vi "Main FPGA.vi"() -> ()   [LabVIEW 2020]
uses:
  <vilib>/Platform/TimedLoop/XDataNode/timing_clust.ctl
  <vilib>/Platform/TimedLoop/XDataNode/nitl_modes.ctl
  <vilib>/Platform/TimedLoop/XDataNode/wakeup.ctl
  <vilib>/rvi/eio/common/nirviEmuTemplateMethod_errors.vi
  <vilib>/rvi/Emulation/niFpgaGetClockAttributes.vi
  <vilib>/rvi/Emulation/niFpgaSctlEmulationGetInTimedLoop.vi
  <vilib>/rvi/Emulation/niFpgaEmulationReportErrorSimple.vi
  <vilib>/rvi/Emulation/niFpgaCriticalErrorInLSC.vi
  <vilib>/rvi/Emulation/niFpgaProcessEmulError.vi
  <vilib>/rvi/interface/RandomDataEmulation/nirviRandomDataMultiElementFPGAFIFO.vi
  <instcachedir>/0/nirviRandomDataMultiElementFPGAFIFO_3E9965BA1FAD4E7B8DABA31768A09B1F.lvgen/nirviRandomDataMultiElementFPGAFIFO_3E9965BA1FAD4E7B8DABA31768A09B1F_001.vi
  <vilib>/rvi/interface/RandomDataEmulation/niFpgaRandomDataHandleErrors.vi
  <vilib>/eio/EIOMethodNode/EIOMethodNode.xnode
  <vilib>/eio/EIONode/EIONode.xnode
  <vilib>/rvi/DataTransferAndStorage/Container/XNode/niFpgaContainer.xnode
  <vilib>/rvi/interface/RandomDataEmulation/nirviRandomDataFpgaMultiElementTemplate.vi
  <vilib>/Platform/TimedLoop/XDataNode/XDataNode.xnode
  <vilib>/Platform/TimedLoop/XDataNode/XDNodeRunTimeDep.lvlib
panel:
  out "Vgen":fxp<+/-,20,5>
  out "Numeric":i32
  out "Timed Out?":bool
  in  "STOP SCTL":bool
  in  "Fase PWM Corrientes":fxp<+,32,0>
  out "Relé encendido":bool
  in  "Fase PWM voltajes":fxp<+,32,0>
  in  "Inc. Fase Volt.":fxp<+,27,0>=0.00020000338554382324
  in  "Freq PWM Corr.":fxp<+,32,0>=0.0005000000819563866
  in  "Freq. PWM Volt.":fxp<+,32,0>=0.0005000000819563866
  in  "Modulacion T002":fxp<+/-,16,1>
  in  "Modulacion T001":fxp<+/-,16,1>
  in  "Factor de Ajuste U1":fxp<+/-,32,2>=1.0
  in  "Factor de Ajuste V1":fxp<+/-,32,2>=0.9900000002235174
  in  "Factor de Ajuste W1":fxp<+/-,32,2>=0.9720000000670552
  in  "Factor de Ajuste U3":fxp<+/-,32,2>=0.9840000001713634
  in  "Factor de Ajuste V3":fxp<+/-,32,2>=0.9840000001713634
  in  "Factor de Ajuste W3":fxp<+/-,32,2>=0.9840000001713634
  out "W4 - U4":fxp<+/-,17,3>
  out "V4 - W4":fxp<+/-,17,3>
  out "U4 - V4":fxp<+/-,17,3>
  out "W3 - U3":fxp<+/-,17,3>
  out "V3 - W3":fxp<+/-,17,3>
  out "U3 - V3":fxp<+/-,17,3>
  out "W2 - U2":fxp<+/-,17,3>
  out "V2 - W2":fxp<+/-,17,3>
  out "U2 - V2":fxp<+/-,17,3>
  out "W1 - U1":fxp<+/-,17,3>
  out "V1 - W1":fxp<+/-,17,3>
  out "U1 - V1":fxp<+/-,17,3>
  in  "Falla U4":bool
  in  "Falla W4":bool
  in  "Falla U3":bool
  in  "Falla W3":bool
  in  "Falla W2":bool
  in  "Falla U2":bool
  in  "Falla W1":bool
  in  "Amplitud Corrientes":fxp<+,32,0>
  in  "Falla U1":bool
  out "sin x + 270":fxp<+/-,16,2>
  out "sin x + 285":fxp<+/-,16,2>
  out "sin x + 165":fxp<+/-,16,2>
  out "sin x + 45":fxp<+/-,16,2>
  out "sin x + 135":fxp<+/-,16,2>
  out "sin x + 150":fxp<+/-,16,2>
  out "sin x + 30":fxp<+/-,16,2>
  out "sin x + 255":fxp<+/-,16,2>
  out "sin x + 15":fxp<+/-,16,2>
  out "sin x + 240":fxp<+/-,16,2>
  out "sin x + 120":fxp<+/-,16,2>
  in  "Phase Inc Corriente":fxp<+,27,0>=0.00010000169277191162
  out "sin(x)":fxp<+/-,16,2>
  in  "Stop While":bool
  out "IExc":fxp<+/-,20,5>
  # "Control PWM de Voltajes"
  # "Importante, para detener la ejecución presionar estos dos botones de STOP"
  # "frecuencia PWM corrientes"
  # "20 kHz / 40 MHz = 0,0005 periods/tick"
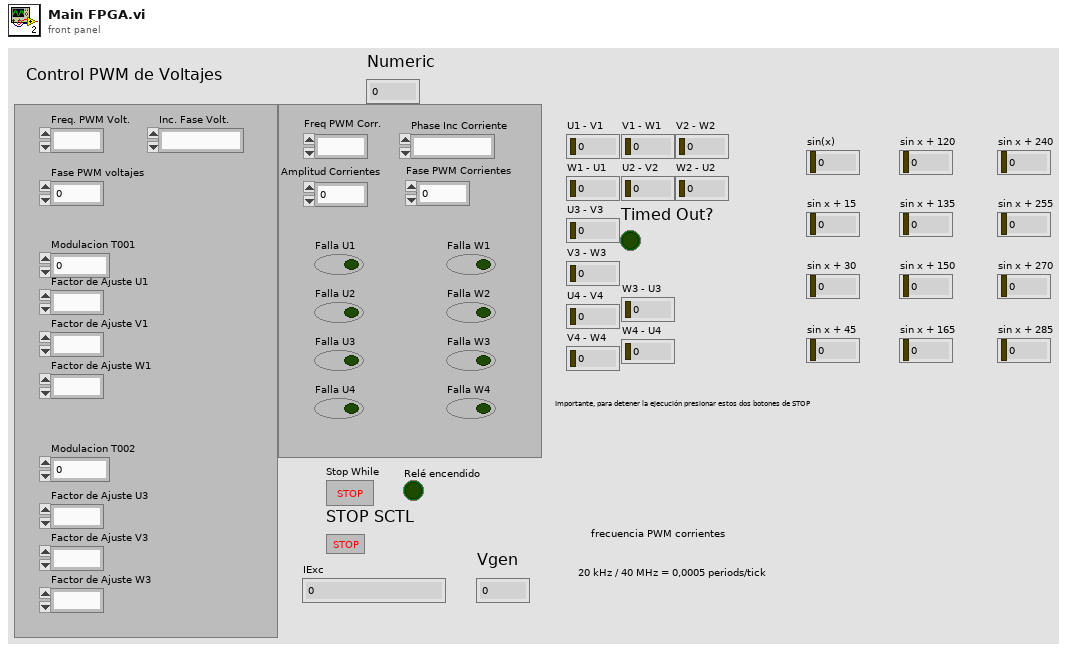
[diagram p1: front panel]
types:
  T1 = typedef "XDNodeRunTimeDep.lvlib/timing_clust.ctl" = cluster{"Expected End [f-1]":u64, "Actual End [f-1]":u64, "Finished Late? [f-1]":bool, "Expected End [i-1]":u64, "Actual End [i-1]":u64, "Finished Late? [i-1]":bool, "Expected Start [i]":u64, "Actual Start [i]":u64, "Expected Start [f]":u64, "Actual Start [f]":u64, "Source Name":string, "Structure Name":string, "Period":i64, "Deadline":i64, "Offset":i64, "Start":i64, "Priority":i32, "Timeout":i32, "Mode":T2, "Wakeup Reason":T3, "Error":errorcluster, "Source Type":string, "Secondary Source Type":string, "Global End Time":u64, "Global Start Time":u64, "Frame Duration":u64, "Iteration Duration":u64, "Assigned CPU":i32, "I/O Scan Engine Mode":u32}
  T2 = typedef "XDNodeRunTimeDep.lvlib/nitl_modes.ctl" = enum32{"No Change", "Process missed periods, maintain original phase", "Discard missed periods, maintain original phase", "Process missed periods, ignore original phase", "Discard missed periods, ignore original phase"}
  T3 = typedef "XDNodeRunTimeDep.lvlib/wakeup.ctl" = enum32{"Normal", "Aborted", "Asynchronous wakeup", "Timing source error", "Timed loop error", "Timeout"}
  T4 = cluster{"U1 - V1":fxp<+/-,17,3>, "V1 - W1":fxp<+/-,17,3>, "W1 - U1":fxp<+/-,17,3>, "U2 - V2":fxp<+/-,17,3>, "V2 - W2":fxp<+/-,17,3>, "W2 - U2":fxp<+/-,17,3>, "U3 - V3":fxp<+/-,17,3>, "V3 - W3":fxp<+/-,17,3>, "W3 - U3":fxp<+/-,17,3>, "U4 - V4":fxp<+/-,17,3>, "V4 - W4":fxp<+/-,17,3>, "W4 - U4":fxp<+/-,17,3>}
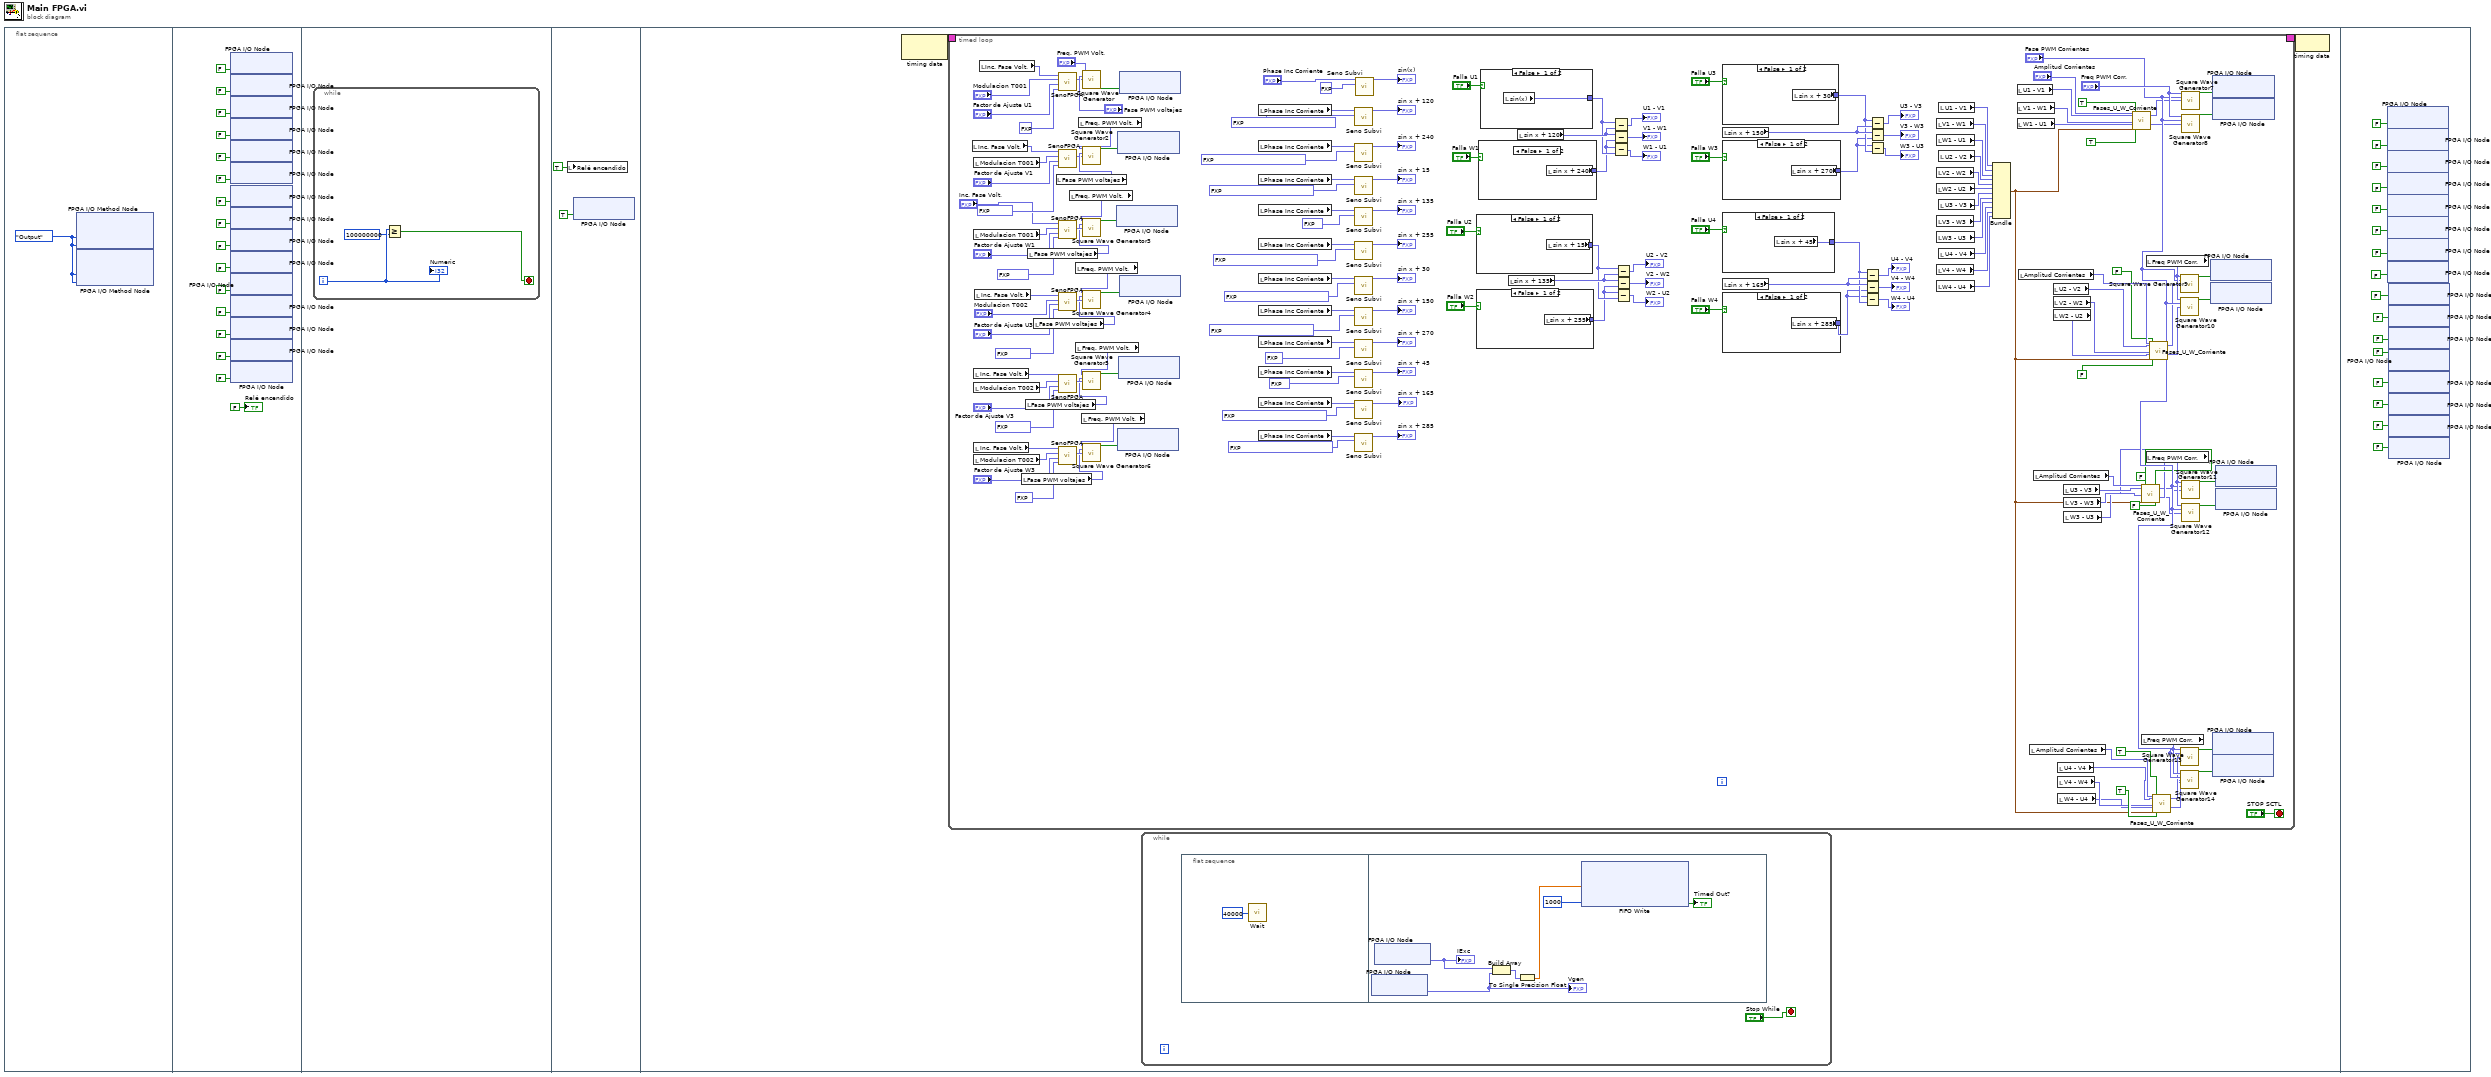
[diagram p0: block diagram]
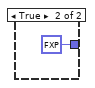
[diagram p2: hidden frame]
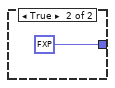
[diagram p3: hidden frame]
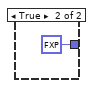
[diagram p4: hidden frame]
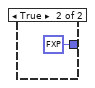
[diagram p5: hidden frame]
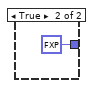
[diagram p6: hidden frame]
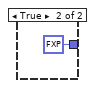
[diagram p7: hidden frame]
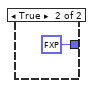
[diagram p8: hidden frame]
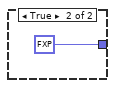
[diagram p9: hidden frame]
diagram:
  n1 = flat-sequence {
    frame #0 {
      w1 = enum8{"No Change", "Input", "Output"}."Output" ("DIO 7:4")
      n2 = xnode "FPGA I/O Method Node"("DIO 7:4"=w1, "DIO 3:0"=w1) -> ()  [unwired: 1 in, 1 out]
      n3 = xnode "FPGA I/O Method Node"("DIO 7:4"=w1, "DIO 3:0"=w1) -> ()  [unwired: 1 in, 1 out]
    }
    frame #1 {
      n4 = xnode "FPGA I/O Node"("Mod1/DIO0"=FALSE) -> ()  [unwired: 1 in, 1 out]
      n5 = xnode "FPGA I/O Node"("Mod1/DIO1"=FALSE) -> ()  [unwired: 1 in, 1 out]
      n6 = xnode "FPGA I/O Node"("Mod1/DIO2"=FALSE) -> ()  [unwired: 1 in, 1 out]
      n7 = xnode "FPGA I/O Node"("Mod1/DIO4"=FALSE ("Mod1/DIO3")) -> ()  [unwired: 1 in, 1 out]
      n8 = xnode "FPGA I/O Node"("Mod1/DIO5"=FALSE ("Mod1/DIO4")) -> ()  [unwired: 1 in, 1 out]
      n9 = xnode "FPGA I/O Node"("Mod1/DIO6"=FALSE ("Mod1/DIO0")) -> ()  [unwired: 1 in, 1 out]
      n10 = xnode "FPGA I/O Node"("Mod1/DIO7"=FALSE ("Mod1/DIO3")) -> ()  [unwired: 1 in, 1 out]
      n11 = xnode "FPGA I/O Node"("Mod2/DIO0"=FALSE ("Mod1/DIO3")) -> ()  [unwired: 1 in, 1 out]
      n12 = xnode "FPGA I/O Node"("Mod2/DIO1"=FALSE ("Mod1/DIO4")) -> ()  [unwired: 1 in, 1 out]
      n13 = xnode "FPGA I/O Node"("Mod2/DIO2"=FALSE ("Mod1/DIO3")) -> ()  [unwired: 1 in, 1 out]
      n14 = xnode "FPGA I/O Node"("Mod2/DIO3"=FALSE ("Mod1/DIO4")) -> ()  [unwired: 1 in, 1 out]
      n15 = xnode "FPGA I/O Node"("Mod2/DIO4"=FALSE ("Mod1/DIO3")) -> ()  [unwired: 1 in, 1 out]
      n16 = xnode "FPGA I/O Node"("Mod2/DIO5"=FALSE ("Mod1/DIO4")) -> ()  [unwired: 1 in, 1 out]
      n17 = xnode "FPGA I/O Node"("Mod2/DIO6"=FALSE ("Mod1/DIO4")) -> ()  [unwired: 1 in, 1 out]
      n18 = xnode "FPGA I/O Node"("Mod2/DIO7"=FALSE ("Mod1/DIO3")) -> ()  [unwired: 1 in, 1 out]
      "Relé encendido" <- FALSE ("Relé encendido")
    }
    frame #2 {
      n19 = while {
        i -> [w20]
        stop <- w18 stop-if-true
        n20 = Greater Or Equal?(x=w20, y=100000000) -> (x >= y?=w18:bool)
        "Numeric" <- w20
      }
    }
    frame #3 {
      n21 = local write "Relé encendido"(TRUE ("Relé encendido")) -> ()
      n22 = xnode "FPGA I/O Node"("Mod1/DIO7"=TRUE ("Mod1/DIO0")) -> ()  [unwired: 1 in, 1 out]
    }
    frame #4 {
      n23 = node-c288() -> (w24:T1)  [unwired: 1 in]
      n24 = timed-loop {
        timing: w24 -> [_]
        timing-out: [_] -> w23
        stop <- "STOP SCTL" stop-if-true
        n25 = local read "Inc. Fase Volt."() -> (w34:fxp<+,27,0>)
        n26 = local read "Modulacion T001"() -> (w110:fxp<+/-,16,1>)
        n27 = local read "Modulacion T001"() -> (w113:fxp<+/-,16,1>)
        n28 = local read "Inc. Fase Volt."() -> (w89:fxp<+,27,0>)
        n29 = local read "Modulacion T002"() -> (w120:fxp<+/-,16,1>)
        n30 = local read "Inc. Fase Volt."() -> (w88:fxp<+,27,0>)
        n31 = local read "Modulacion T002"() -> (w124:fxp<+/-,16,1>)
        n32 = local read "Inc. Fase Volt."() -> (w90:fxp<+,27,0>)
        n33 = local read "Inc. Fase Volt."() -> (w35:fxp<+,27,0>)
        n34 = local read "Fase PWM voltajes"() -> (w74:fxp<+,32,0>)
        n35 = local read "Fase PWM voltajes"() -> (w75:fxp<+,32,0>)
        n36 = local read "Fase PWM voltajes"() -> (w77:fxp<+,32,0>)
        n37 = local read "Fase PWM voltajes"() -> (w76:fxp<+,32,0>)
        n38 = local read "Fase PWM voltajes"() -> (w78:fxp<+,32,0>)
        n39 = call "SenoFPGA.vi"("Fase Inicial"=fxp<+,27,1> 0.0 ("Fase Inicial U1"), "Factor de Ajuste"="Factor de Ajuste U1", "Modulacion T001"="Modulacion T001", "Tasa de Incremento de Fase"=w35) -> ("Sine Wave"=w38:fxp<+/-,32,2>)  [unwired: 7 in]
        n40 = call "SenoFPGA.vi"("Fase Inicial"=fxp<+,27,1> 0.6666666567325592 ("Fase Inicial V1"), "Factor de Ajuste"="Factor de Ajuste V1", "Modulacion T001"=w110, "Tasa de Incremento de Fase"=w34) -> ("Sine Wave"=w37:fxp<+/-,32,2>)  [unwired: 7 in]
        n41 = call "SenoFPGA.vi"("Fase Inicial"=fxp<+,27,1> 1.3333333283662796 ("Fase Inicial W1"), "Factor de Ajuste"="Factor de Ajuste W1", "Modulacion T001"=w113, "Tasa de Incremento de Fase"="Inc. Fase Volt.") -> ("Sine Wave"=w114:fxp<+/-,32,2>)  [unwired: 7 in]
        n42 = call "SenoFPGA.vi"("Fase Inicial"=fxp<+,27,1> 0.16666659712791443 ("Fase Inicial U3"), "Factor de Ajuste"="Factor de Ajuste U3", "Modulacion T001"="Modulacion T002", "Tasa de Incremento de Fase"=w90) -> ("Sine Wave"=w117:fxp<+/-,32,2>)  [unwired: 7 in]
        n43 = call "SenoFPGA.vi"("Fase Inicial"=fxp<+,27,1> 0.8333333283662796 ("Fase Inicial V3"), "Factor de Ajuste"="Factor de Ajuste V3", "Modulacion T001"=w120, "Tasa de Incremento de Fase"=w89) -> ("Sine Wave"=w121:fxp<+/-,32,2>)  [unwired: 7 in]
        n44 = call "SenoFPGA.vi"("Fase Inicial"=fxp<+,27,1> 1.5 ("Fase Inicial W3"), "Factor de Ajuste"="Factor de Ajuste W3", "Modulacion T001"=w124, "Tasa de Incremento de Fase"=w88) -> ("Sine Wave"=w125:fxp<+/-,32,2>)  [unwired: 7 in]
        n45 = local read "Freq. PWM Volt."() -> (w99:fxp<+,32,0>)
        n46 = local read "Freq. PWM Volt."() -> (w98:fxp<+,32,0>)
        n47 = local read "Freq. PWM Volt."() -> (w97:fxp<+,32,0>)
        n48 = local read "Freq. PWM Volt."() -> (w100:fxp<+,32,0>)
        n49 = local read "Freq. PWM Volt."() -> (w96:fxp<+,32,0>)
        n50 = call "Square Wave Generator"("frequency (periods/tick)"="Freq. PWM Volt.", "phase offset (periods)"="Fase PWM voltajes", "duty cycle (periods)"=w38) -> ("square wave out"=w107:bool)  [unwired: 12 in]
        n51 = call "Square Wave Generator2"("frequency (periods/tick)"=w100, "phase offset (periods)"=w78, "duty cycle (periods)"=w37) -> ("square wave out"=w106:bool)  [unwired: 12 in]
        n52 = call "Square Wave Generator3"("frequency (periods/tick)"=w99, "phase offset (periods)"=w77, "duty cycle (periods)"=w114) -> ("square wave out"=w105:bool)  [unwired: 12 in]
        n53 = call "Square Wave Generator4"("frequency (periods/tick)"=w98, "phase offset (periods)"=w76, "duty cycle (periods)"=w117) -> ("square wave out"=w104:bool)  [unwired: 12 in]
        n54 = call "Square Wave Generator5"("frequency (periods/tick)"=w97, "phase offset (periods)"=w75, "duty cycle (periods)"=w121) -> ("square wave out"=w103:bool)  [unwired: 12 in]
        n55 = call "Square Wave Generator6"("frequency (periods/tick)"=w96, "phase offset (periods)"=w74, "duty cycle (periods)"=w125) -> ("square wave out"=w102:bool)  [unwired: 12 in]
        n56 = xnode "FPGA I/O Node"("Mod1/DIO2"=w105) -> ()  [unwired: 1 in, 1 out]
        n57 = xnode "FPGA I/O Node"("Mod1/DIO6"=w102) -> ()  [unwired: 1 in, 1 out]
        n58 = xnode "FPGA I/O Node"("Mod1/DIO1"=w106) -> ()  [unwired: 1 in, 1 out]
        n59 = xnode "FPGA I/O Node"("Mod1/DIO5"=w103) -> ()  [unwired: 1 in, 1 out]
        n60 = xnode "FPGA I/O Node"("Mod1/DIO0"=w107) -> ()  [unwired: 1 in, 1 out]
        n61 = xnode "FPGA I/O Node"("Mod1/DIO4"=w104) -> ()  [unwired: 1 in, 1 out]
        n62 = local read "Phase Inc Corriente"() -> (w206:fxp<+,27,0>)
        n63 = local read "Phase Inc Corriente"() -> (w205:fxp<+,27,0>)
        n64 = local read "Phase Inc Corriente"() -> (w204:fxp<+,27,0>)
        n65 = local read "Phase Inc Corriente"() -> (w200:fxp<+,27,0>)
        n66 = local read "Phase Inc Corriente"() -> (w201:fxp<+,27,0>)
        n67 = local read "Phase Inc Corriente"() -> (w202:fxp<+,27,0>)
        n68 = local read "Phase Inc Corriente"() -> (w203:fxp<+,27,0>)
        n69 = local read "Phase Inc Corriente"() -> (w196:fxp<+,27,0>)
        n70 = local read "Phase Inc Corriente"() -> (w197:fxp<+,27,0>)
        n71 = local read "Phase Inc Corriente"() -> (w198:fxp<+,27,0>)
        n72 = local read "Phase Inc Corriente"() -> (w199:fxp<+,27,0>)
        n73 = call "Seno Subvi.vi"("Fase Inicial"=fxp<+,27,1> 0.6666666716337204, "Phase Inc Corriente"=w206) -> ("sin(x)"=→"sin x + 120":fxp<+/-,16,2>)  [unwired: 9 in]
        n74 = call "Seno Subvi.vi"("Fase Inicial"=fxp<+,27,1> 1.3333333283662796 ("control fase"), "Phase Inc Corriente"=w205) -> ("sin(x)"=→"sin x + 240":fxp<+/-,16,2>)  [unwired: 9 in]
        n75 = call "Seno Subvi.vi"("Fase Inicial"=fxp<+,27,1> 0.0833333283662796 ("control fase"), "Phase Inc Corriente"=w204) -> ("sin(x)"=→"sin x + 15":fxp<+/-,16,2>)  [unwired: 9 in]
        n76 = call "Seno Subvi.vi"("Fase Inicial"=fxp<+,27,1> 0.75 ("control fase"), "Phase Inc Corriente"=w200) -> ("sin(x)"=→"sin x + 135":fxp<+/-,16,2>)  [unwired: 9 in]
        n77 = call "Seno Subvi.vi"("Fase Inicial"=fxp<+,27,1> 1.4166666716337204 ("control fase"), "Phase Inc Corriente"=w201) -> ("sin(x)"=→"sin x + 255":fxp<+/-,16,2>)  [unwired: 9 in]
        n78 = call "Seno Subvi.vi"("Fase Inicial"=fxp<+,27,1> 0.1666666716337204 ("control fase"), "Phase Inc Corriente"=w202) -> ("sin(x)"=→"sin x + 30":fxp<+/-,16,2>)  [unwired: 9 in]
        n79 = call "Seno Subvi.vi"("Fase Inicial"=fxp<+,27,1> 0.8333333283662796 ("control fase"), "Phase Inc Corriente"=w203) -> ("sin(x)"=→"sin x + 150":fxp<+/-,16,2>)  [unwired: 9 in]
        n80 = call "Seno Subvi.vi"("Fase Inicial"=fxp<+,27,1> 1.5 ("control fase"), "Phase Inc Corriente"=w196) -> ("sin(x)"=→"sin x + 270":fxp<+/-,16,2>)  [unwired: 9 in]
        n81 = call "Seno Subvi.vi"("Fase Inicial"=fxp<+,27,1> 0.25 ("control fase"), "Phase Inc Corriente"=w197) -> ("sin(x)"=→"sin x + 45":fxp<+/-,16,2>)  [unwired: 9 in]
        n82 = call "Seno Subvi.vi"("Fase Inicial"=fxp<+,27,1> 0.9166666716337204 ("control fase"), "Phase Inc Corriente"=w198) -> ("sin(x)"=→"sin x + 165":fxp<+/-,16,2>)  [unwired: 9 in]
        n83 = call "Seno Subvi.vi"("Fase Inicial"=fxp<+,27,1> 1.5833333283662796 ("control fase"), "Phase Inc Corriente"=w199) -> ("sin(x)"=→"sin x + 285":fxp<+/-,16,2>)  [unwired: 9 in]
        n84 = call "Seno Subvi.vi"("Fase Inicial"=fxp<+,27,1> 0.0, "Phase Inc Corriente"="Phase Inc Corriente") -> ("sin(x)"=→"sin(x)":fxp<+/-,16,2>)  [unwired: 9 in]
        n85 = case shown="False" "Falla W2" {
          tunnel: [w216 fxp<+/-,16,2> 0.0 ("sin(x)")] -> w160
          frame False {
            n86 = local read "sin x + 255"() -> (w216:fxp<+/-,16,2>)
          }
          frame True {
          }
        }
        n87 = case shown="False" "Falla U2" {
          tunnel: [w218 fxp<+/-,16,2> 0.0 ("sin(x)")] -> w162
          frame False {
            n88 = local read "sin x + 15"() -> (w218:fxp<+/-,16,2>)
          }
          frame True {
          }
        }
        n89 = case shown="False" "Falla W1" {
          tunnel: [w220 fxp<+/-,16,2> 0.0 ("sin(x)")] -> w95
          frame False {
            n90 = local read "sin x + 240"() -> (w220:fxp<+/-,16,2>)
          }
          frame True {
          }
        }
        n91 = case shown="False" "Falla U1" {
          tunnel: [w222 fxp<+/-,16,2> 0.0 ("sin(x)")] -> w168
          frame False {
            n92 = local read "sin(x)"() -> (w222:fxp<+/-,16,2>)
          }
          frame True {
          }
        }
        n93 = local read "sin x + 135"() -> (w172:fxp<+/-,16,2>)
        n94 = local read "sin x + 120"() -> (w169:fxp<+/-,16,2>)
        n95 = Subtract(x=w168, y=w169) -> (x-y=→"U1 - V1":fxp<+/-,17,3>)
        n96 = Subtract(x=w169, y=w95) -> (x-y=→"V1 - W1":fxp<+/-,17,3>)
        n97 = Subtract(x=w95, y=w168) -> (x-y=→"W1 - U1":fxp<+/-,17,3>)
        n98 = Subtract(x=w162, y=w172) -> (x-y=→"U2 - V2":fxp<+/-,17,3>)
        n99 = Subtract(x=w172, y=w160) -> (x-y=→"V2 - W2":fxp<+/-,17,3>)
        n100 = Subtract(x=w160, y=w162) -> (x-y=→"W2 - U2":fxp<+/-,17,3>)
        n101 = case shown="False" "Falla U3" {
          tunnel: [w214 fxp<+/-,16,2> 0.0 ("sin(x)")] -> w157
          frame False {
            n102 = local read "sin x + 30"() -> (w214:fxp<+/-,16,2>)
          }
          frame True {
          }
        }
        n103 = local read "sin x + 150"() -> (w171:fxp<+/-,16,2>)
        n104 = case shown="False" "Falla W3" {
          tunnel: [w212 fxp<+/-,16,2> 0.0 ("sin(x)")] -> w156
          frame False {
            n105 = local read "sin x + 270"() -> (w212:fxp<+/-,16,2>)
          }
          frame True {
          }
        }
        n106 = case shown="False" "Falla U4" {
          tunnel: [w210 fxp<+/-,16,2> 0.0 ("sin(x)")] -> w153
          frame False {
            n107 = local read "sin x + 45"() -> (w210:fxp<+/-,16,2>)
          }
          frame True {
          }
        }
        n108 = local read "sin x + 165"() -> (w170:fxp<+/-,16,2>)
        n109 = case shown="False" "Falla W4" {
          tunnel: [w208 fxp<+/-,16,2> 0.0 ("sin(x)")] -> w152
          frame False {
            n110 = local read "sin x + 285"() -> (w208:fxp<+/-,16,2>)
          }
          frame True {
          }
        }
        n111 = Subtract(x=w153, y=w170) -> (x-y=→"U4 - V4":fxp<+/-,17,3>)
        n112 = Subtract(x=w170, y=w152) -> (x-y=→"V4 - W4":fxp<+/-,17,3>)
        n113 = Subtract(x=w152, y=w153) -> (x-y=→"W4 - U4":fxp<+/-,17,3>)
        n114 = Subtract(x=w157, y=w171) -> (x-y=→"U3 - V3":fxp<+/-,17,3>)
        n115 = Subtract(x=w171, y=w156) -> (x-y=→"V3 - W3":fxp<+/-,17,3>)
        n116 = Subtract(x=w156, y=w157) -> (x-y=→"W3 - U3":fxp<+/-,17,3>)
        n117 = local read "V1 - W1"() -> (w144:fxp<+/-,17,3>)
        n118 = local read "W1 - U1"() -> (w143:fxp<+/-,17,3>)
        n119 = local read "V2 - W2"() -> (w141:fxp<+/-,17,3>)
        n120 = local read "W2 - U2"() -> (w140:fxp<+/-,17,3>)
        n121 = local read "V3 - W3"() -> (w138:fxp<+/-,17,3>)
        n122 = local read "W3 - U3"() -> (w137:fxp<+/-,17,3>)
        n123 = local read "V4 - W4"() -> (w135:fxp<+/-,17,3>)
        n124 = local read "W4 - U4"() -> (w134:fxp<+/-,17,3>)
        n125 = local read "U1 - V1"() -> (w129:fxp<+/-,17,3>)
        n126 = local read "U2 - V2"() -> (w142:fxp<+/-,17,3>)
        n127 = local read "U3 - V3"() -> (w139:fxp<+/-,17,3>)
        n128 = local read "U4 - V4"() -> (w136:fxp<+/-,17,3>)
        n129 = Bundle("U1 - V1"=w129, "V1 - W1"=w144, "W1 - U1"=w143, "U2 - V2"=w142, "V2 - W2"=w141, "W2 - U2"=w140, "U3 - V3"=w139, "V3 - W3"=w138, "W3 - U3"=w137, "U4 - V4"=w136, "V4 - W4"=w135, "W4 - U4"=w134) -> (w42:T4)  [unwired: 1 in]
        n130 = local read "U1 - V1"() -> (w71:fxp<+/-,17,3>)
        n131 = local read "V1 - W1"() -> (w70:fxp<+/-,17,3>)
        n132 = local read "W1 - U1"() -> (w69:fxp<+/-,17,3>)
        n133 = local read "Amplitud Corrientes"() -> (w64:fxp<+,32,0>)
        n134 = local read "Amplitud Corrientes"() -> (w46:fxp<+,32,0>)
        n135 = local read "Amplitud Corrientes"() -> (w54:fxp<+,32,0>)
        n136 = local read "U2 - V2"() -> (w63:fxp<+/-,17,3>)
        n137 = local read "V2 - W2"() -> (w62:fxp<+/-,17,3>)
        n138 = local read "W2 - U2"() -> (w61:fxp<+/-,17,3>)
        n139 = local read "U4 - V4"() -> (w45:fxp<+/-,17,3>)
        n140 = local read "V4 - W4"() -> (w44:fxp<+/-,17,3>)
        n141 = local read "W4 - U4"() -> (w43:fxp<+/-,17,3>)
        n142 = local read "U3 - V3"() -> (w53:fxp<+/-,17,3>)
        n143 = local read "V3 - W3"() -> (w52:fxp<+/-,17,3>)
        n144 = local read "W3 - U3"() -> (w51:fxp<+/-,17,3>)
        n145 = call "Fases_U_W_Corriente.vi"("Amplitud Corrientes"="Amplitud Corrientes", "U-V"=w71, "V-W"=w70, "W-U"=w69, "Cluster Diferencia de Voltajes"=w42, "Polaridad L-K en U?"=TRUE ("U L-K?"), "Polaridad L-K en W?"=TRUE ("W L-K?")) -> ("Pulsos Corriente U"=w68:fxp<+/-,34,2>, "Pulsos Corriente W"=w67:fxp<+/-,34,2>)  [unwired: 19 in]
        n146 = local read "Freq PWM Corr."() -> (w91:fxp<+,32,0>)
        n147 = call "Fases_U_W_Corriente.vi"("Amplitud Corrientes"=w54, "U-V"=w53, "V-W"=w52, "W-U"=w51, "Cluster Diferencia de Voltajes"=w42, "Polaridad L-K en U?"=FALSE ("U L-K? 3"), "Polaridad L-K en W?"=FALSE ("W L-K? 3")) -> ("Pulsos Corriente U"=w50:fxp<+/-,34,2>, "Pulsos Corriente W"=w49:fxp<+/-,34,2>)  [unwired: 19 in]
        n148 = local read "Freq PWM Corr."() -> (w93:fxp<+,32,0>)
        n149 = local read "Freq PWM Corr."() -> (w92:fxp<+,32,0>)
        n150 = call "Fases_U_W_Corriente.vi"("Amplitud Corrientes"=w64, "U-V"=w63, "V-W"=w62, "W-U"=w61, "Cluster Diferencia de Voltajes"=w42, "Polaridad L-K en U?"=FALSE ("U L-K? 2"), "Polaridad L-K en W?"=FALSE) -> ("Pulsos Corriente U"=w60:fxp<+/-,34,2>, "Pulsos Corriente W"=w59:fxp<+/-,34,2>)  [unwired: 19 in]
        n151 = call "Fases_U_W_Corriente.vi"("Amplitud Corrientes"=w46, "U-V"=w45, "V-W"=w44, "W-U"=w43, "Cluster Diferencia de Voltajes"=w42, "Polaridad L-K en U?"=TRUE ("U L-K? 4"), "Polaridad L-K en W?"=TRUE ("W L-K? 4")) -> ("Pulsos Corriente U"=w41:fxp<+/-,34,2>, "Pulsos Corriente W"=w40:fxp<+/-,34,2>)  [unwired: 19 in]
        n152 = call "Square Wave Generator9"("frequency (periods/tick)"=w93, "phase offset (periods)"="Fase PWM Corrientes", "duty cycle (periods)"=w60) -> ("square wave out"=w85:bool)  [unwired: 12 in]
        n153 = call "Square Wave Generator10"("frequency (periods/tick)"=w93, "phase offset (periods)"="Fase PWM Corrientes", "duty cycle (periods)"=w59) -> ("square wave out"=w84:bool)  [unwired: 12 in]
        n154 = call "Square Wave Generator13"("frequency (periods/tick)"=w91, "phase offset (periods)"="Fase PWM Corrientes", "duty cycle (periods)"=w41) -> ("square wave out"=w81:bool)  [unwired: 12 in]
        n155 = call "Square Wave Generator14"("frequency (periods/tick)"=w91, "phase offset (periods)"="Fase PWM Corrientes", "duty cycle (periods)"=w40) -> ("square wave out"=w80:bool)  [unwired: 12 in]
        n156 = call "Square Wave Generator7"("frequency (periods/tick)"="Freq PWM Corr.", "phase offset (periods)"="Fase PWM Corrientes", "duty cycle (periods)"=w68) -> ("square wave out"=w87:bool)  [unwired: 12 in]
        n157 = call "Square Wave Generator8"("frequency (periods/tick)"="Freq PWM Corr.", "phase offset (periods)"="Fase PWM Corrientes", "duty cycle (periods)"=w67) -> ("square wave out"=w86:bool)  [unwired: 12 in]
        n158 = call "Square Wave Generator11"("frequency (periods/tick)"=w92, "phase offset (periods)"="Fase PWM Corrientes", "duty cycle (periods)"=w50) -> ("square wave out"=w83:bool)  [unwired: 12 in]
        n159 = call "Square Wave Generator12"("frequency (periods/tick)"=w92, "phase offset (periods)"="Fase PWM Corrientes", "duty cycle (periods)"=w49) -> ("square wave out"=w82:bool)  [unwired: 12 in]
        n160 = xnode "FPGA I/O Node"("Mod2/DIO2"=w85) -> ()  [unwired: 1 in, 1 out]
        n161 = xnode "FPGA I/O Node"("Mod2/DIO3"=w84) -> ()  [unwired: 1 in, 1 out]
        n162 = xnode "FPGA I/O Node"("Mod2/DIO6"=w81) -> ()  [unwired: 1 in, 1 out]
        n163 = xnode "FPGA I/O Node"("Mod2/DIO7"=w80) -> ()  [unwired: 1 in, 1 out]
        n164 = xnode "FPGA I/O Node"("Mod2/DIO0"=w87) -> ()  [unwired: 1 in, 1 out]
        n165 = xnode "FPGA I/O Node"("Mod2/DIO1"=w86) -> ()  [unwired: 1 in, 1 out]
        n166 = xnode "FPGA I/O Node"("Mod2/DIO4"=w83) -> ()  [unwired: 1 in, 1 out]
        n167 = xnode "FPGA I/O Node"("Mod2/DIO5"=w82) -> ()  [unwired: 1 in, 1 out]
      }
      n168 = while {
        stop <- "Stop While" stop-if-true
        n169 = flat-sequence {
          frame #0 {
            n170 = call "Wait"("Count(Ticks)"=u32 40000) -> ()  [unwired: 1 out]
          }
          frame #1 {
            n171 = xnode "FPGA I/O Node"() -> ("Mod3/AI1"=w27:fxp<+/-,20,5>)  [unwired: 1 in, 1 out]
            "Vgen" <- w27
            n172 = xnode "FPGA I/O Node"() -> ("Mod3/AI0"=w29:fxp<+/-,20,5>)  [unwired: 1 in, 1 out]
            "IExc" <- w29
            n173 = Build Array(w29, w27) -> (w30:fxp<+/-,20,5>[])
            n174 = To Single Precision Float(number=w30) -> (single precision float=w31:sgl[])
            n175 = xnode ("FIFO Write")("Element"=w31, "Timeout"=1000) -> ("Timed Out?"=→"Timed Out?":bool)  [unwired: 1 in, 1 out]
          }
        }
      }
      n176 = node-c288(w23) -> ()
    }
    frame #5 {
      n177 = xnode "FPGA I/O Node"("Mod1/DIO0"=FALSE) -> ()  [unwired: 1 in, 1 out]
      n178 = xnode "FPGA I/O Node"("Mod1/DIO1"=FALSE) -> ()  [unwired: 1 in, 1 out]
      n179 = xnode "FPGA I/O Node"("Mod1/DIO2"=FALSE) -> ()  [unwired: 1 in, 1 out]
      n180 = xnode "FPGA I/O Node"("Mod1/DIO3"=FALSE) -> ()  [unwired: 1 in, 1 out]
      n181 = xnode "FPGA I/O Node"("Mod1/DIO4"=FALSE) -> ()  [unwired: 1 in, 1 out]
      n182 = xnode "FPGA I/O Node"("Mod1/DIO5"=FALSE ("Mod1/DIO0")) -> ()  [unwired: 1 in, 1 out]
      n183 = xnode "FPGA I/O Node"("Mod1/DIO6"=FALSE ("Mod1/DIO1")) -> ()  [unwired: 1 in, 1 out]
      n184 = xnode "FPGA I/O Node"("Mod1/DIO7"=FALSE ("Mod1/DIO2")) -> ()  [unwired: 1 in, 1 out]
      n185 = xnode "FPGA I/O Node"("Mod2/DIO1"=FALSE ("Mod1/DIO4")) -> ()  [unwired: 1 in, 1 out]
      n186 = xnode "FPGA I/O Node"("Mod2/DIO0"=FALSE ("Mod1/DIO3")) -> ()  [unwired: 1 in, 1 out]
      n187 = xnode "FPGA I/O Node"("Mod2/DIO2"=FALSE ("Mod1/DIO3")) -> ()  [unwired: 1 in, 1 out]
      n188 = xnode "FPGA I/O Node"("Mod2/DIO3"=FALSE ("Mod1/DIO4")) -> ()  [unwired: 1 in, 1 out]
      n189 = xnode "FPGA I/O Node"("Mod2/DIO4"=FALSE ("Mod1/DIO3")) -> ()  [unwired: 1 in, 1 out]
      n190 = xnode "FPGA I/O Node"("Mod2/DIO5"=FALSE ("Mod1/DIO4")) -> ()  [unwired: 1 in, 1 out]
      n191 = xnode "FPGA I/O Node"("Mod2/DIO6"=FALSE ("Mod1/DIO3")) -> ()  [unwired: 1 in, 1 out]
      n192 = xnode "FPGA I/O Node"("Mod2/DIO7"=FALSE ("Mod1/DIO4")) -> ()  [unwired: 1 in, 1 out]
    }
  }
